vi "Main.vi"(8 "error in (no error)":errorcluster) -> (0 "error out":errorcluster)   [LabVIEW 2017]
doc: "Main application that is run to test ATM algorithms."
uses:
  Controller/Controls/Interface.ctl
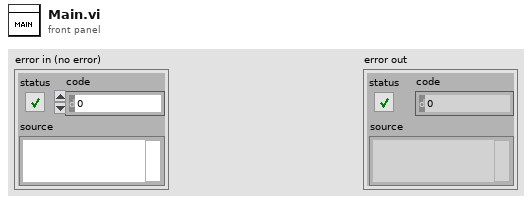
[diagram p1: front panel]
types:
  T1 = typedef "UE Data Container.ctl" = cluster{"Stop UE":refnum<user-event>, "Error UE":refnum<user-event>, "Deposit Change":refnum<user-event>, "Funds Change":refnum<user-event>, "Card Reader Change":refnum<user-event>, "Transaction Change":refnum<user-event>, "Keypad Screen Change":refnum<user-event>}
  T2 = typedef "Queues.ctl" = cluster{"Controller":refnum<queue>, "Config":refnum<queue>, "Display Console":refnum<queue>}
  T3 = typedef "Interface.ctl" = enum16{"Simulated", "Hardware"}
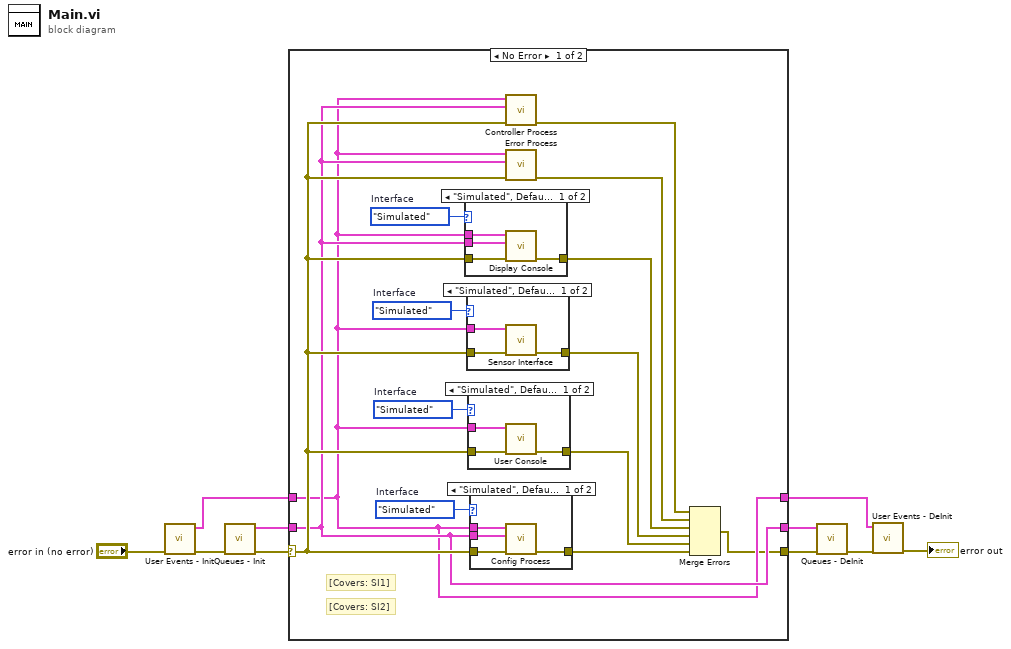
[diagram p0: block diagram]
diagram:
  n1 = call "User Events - Init.vi"("error in (no error)"="error in (no error)") -> ("error out"=w9:errorcluster, "UE Data Container"=w7:T1)  [unwired: 9 in]
  n2 = call "Queues - Init.vi"("error in (no error)"=w9) -> ("error out"=w8:errorcluster, "Queues"=w6:T2)  [unwired: 9 in]
  n3 = case shown="No Error" w8 {
    selector: w8 -> [w20 w43]
    tunnel: w7 -> [w18 w45]
    tunnel: w6 -> [w19 w44]
    tunnel: [w18 w45] -> w2
    tunnel: [w19 w44] -> w4
    tunnel: [w11 w43] -> w5
    frame No Error {
      w21 = Interface."Simulated"  # Interface
      w22 = Interface."Simulated"  # Interface
      w23 = Interface."Simulated"  # Interface
      w24 = Interface."Simulated"  # Interface
      # "[Covers: SI2]"
      # "[Covers: SI1]"
      n4 = case shown="\"Simulated\", Default" w21 {
        tunnel: w20 -> [w27 w29]
        tunnel: [w28 w29] -> w14
        tunnel: w19 -> [w26 _]
        tunnel: w18 -> [w25 _]
        frame "Simulated", Default {
          n5 = call "Display Console.vi"("error in (no error)"=w27, "Queues"=w26, "UE Data Container"=w25) -> ("error out"=w28:errorcluster)  [unwired: 8 in]
        }
        frame "Hardware" {
        }
      }
      n6 = case shown="\"Simulated\", Default" w22 {
        tunnel: w20 -> [w31 w33]
        tunnel: [w32 w33] -> w15
        tunnel: w18 -> [w30 _]
        frame "Simulated", Default {
          n7 = call "Sensor Interface.vi"("error in (no error)"=w31, "UE Data Container"=w30) -> ("error out"=w32:errorcluster)  [unwired: 9 in]
        }
        frame "Hardware" {
        }
      }
      n8 = case shown="\"Simulated\", Default" w23 {
        tunnel: w20 -> [w35 w37]
        tunnel: [w36 w37] -> w16
        tunnel: w18 -> [w34 _]
        frame "Simulated", Default {
          n9 = call "User Console.vi"("error in (no error)"=w35, "UE Data Container"=w34) -> ("error out"=w36:errorcluster)  [unwired: 9 in]
        }
        frame "Hardware" {
        }
      }
      n10 = case shown="\"Simulated\", Default" w24 {
        tunnel: w20 -> [w41 w42]
        tunnel: [w40 w42] -> w17
        tunnel: w19 -> [w39 _]
        tunnel: w18 -> [w38 _]
        frame "Simulated", Default {
          n11 = call "Config Process.vi"("error in (no error)"=w41, "Queues"=w39, "UE Data Container"=w38) -> ("error out"=w40:errorcluster)  [unwired: 8 in]
        }
        frame "Hardware" {
        }
      }
      n12 = call "Controller Process.vi"("error in (no error)"=w20, "Queues"=w19, "UE Data Container"=w18) -> ("error out"=w12:errorcluster)  [unwired: 8 in]
      n13 = call "Error Process.vi"("error in (no error)"=w20, "Queues"=w19, "UE Data Container"=w18) -> ("error out"=w13:errorcluster)  [unwired: 8 in]
      n14 = Merge Errors(w12, w13, w14, w15, w16, w17) -> (w11:errorcluster)
    }
    frame Error {
    }
  }
  n15 = call "Queues - DeInit.vi"("error in (no error)"=w5, "Queues"=w4) -> ("error out"=w3:errorcluster)  [unwired: 9 in]
  n16 = call "User Events - DeInit.vi"("error in (no error)"=w3, "UE Data Container"=w2) -> ("error out"=→"error out":errorcluster)  [unwired: 9 in]
